vi "Choice.vi"(9 "g":u32 format="0x%08x", 10 "f":u32 format="0x%08x", 11 "e":u32 format="0x%08x") -> (2 "Ch":u32 format="0x%08x")   [LabVIEW 2020, in "Crypto.lvlib" / "SHA-256.lvclass"]
uses:
  SHA-256.lvclass
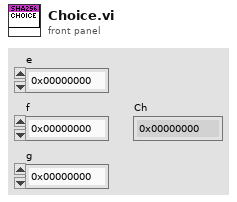
[diagram p1: front panel]
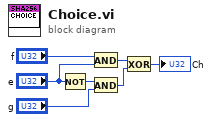
[diagram p0: block diagram]
diagram:
  n1 = Not(x="e") -> (.not. x?=w5:u32)
  n2 = And(x="f", y="e") -> (x .and. y?=w7:u32)
  n3 = And(x=w5, y="g") -> (x .and. y?=w6:u32)
  n4 = Exclusive Or(1:w6, 2:w7) -> (0:→"Ch":u32)
